vi "ziExample-Module-DAQ_triggerUtility.vi"() -> ()   [LabVIEW 2009]
doc: "Control a Zurich instrument device via the LabOne Labview API. \nRequirements: Zurich Instruments MFLI, HF2 or UHFLI \nThis example shows how to start a DAQ trigger module and retrieve the Data.\n\n© Zurich Instruments AG, www.zhinst.com"
uses:
  <instrlib>/Zurich Instruments LabOne/Public/Modules/ziTypeModEnum.ctl
  <instrlib>/Zurich Instruments LabOne/Public/Modules/ziModSetValueBinary.vi
  <instrlib>/Zurich Instruments LabOne/Public/Configure/ziSetValueDoubleArray.vi
  <instrlib>/Zurich Instruments LabOne/Public/Modules/ziModSetValueDouble.vi
  <instrlib>/Zurich Instruments LabOne/Public/Modules/ziModGetDoubleData.vi
  <instrlib>/Zurich Instruments LabOne/Public/Utility/ziTicksToS_vector.vi
  <instrlib>/Zurich Instruments LabOne/Public/Utility/ziTicksToS_single.vi
  <instrlib>/Zurich Instruments LabOne/Zurich Instruments LabOne.lvlib
panel:
  in  "beating":bool caption="Beating (needs MD/MF Option)"
  out "Slide":dbl(slide) scale=0.0..1.0
  in  "subscribe":string="demods/0/sample.R.avg"
  out "Grid DEMOD X":dbl[][](graph)
  out "Error Out":errorcluster
  in  "stop":bool
  in  "run":bool caption="Run"
  in  "TriggerModulSetup":T1={"holdoff/time"=0.2, "holdoff/count"=0.0, "delay"=-0.00125, "duration"=0.01, "pulse/min"=0.0, "pulse/max"=0.0, "type"=1, "edge"=1, "count"=5.0, "bits"=1.0, "bitmask"=1.0, "triggernode"="demods/0/sample.R", "bandwidth"=0.0, "hysteresis"=0.003, "level"=0.03, "grid/mode"=1.0, "grid/cols"=100, "grid/rows"=100, "grid/direction"=0.0, "grid/repetitions"=1.0} {"grid/direction" items=["Forward", "Reverse", "Bi-directional"]; "grid/mode" items=["OFF", "Nearest", "Linear"]; "level" format="%#_6p"; "hysteresis" format="%#_6p"; "bandwidth" format="%#_6p"; "edge" items=["positive"=1, "negative"=2, "both"=3]; "type" items=["edge"=1, "digital"=2, "pulse"=3, "tracking edge"=4, "HW Trigger"=6, "tracking pulse"=7]}
  out "Demod X":T2(graph)
  in  "Address":string="DEV"
  out "Selected Device":string
  # "ziExample-Module-DAQ_triggerUtility.vi\nRequirements: \n- HF2LI, UHFLI or MFLI \n- MD Option\nsee block diagram for VI description"
  # "Tested Instruments:\n- HF2LI\n- UHFLI\n- MFLI"
  # "Trigger Settings"
  # "edge/pulse/tracking edge/tracking pulse"
  # "only for tracking mode"
  # "digital"
  # "Horizontal"
  # "only for pulse/tracking pulse"
  # "only for pulse/tracking pulse"
  # "Grid Mode"
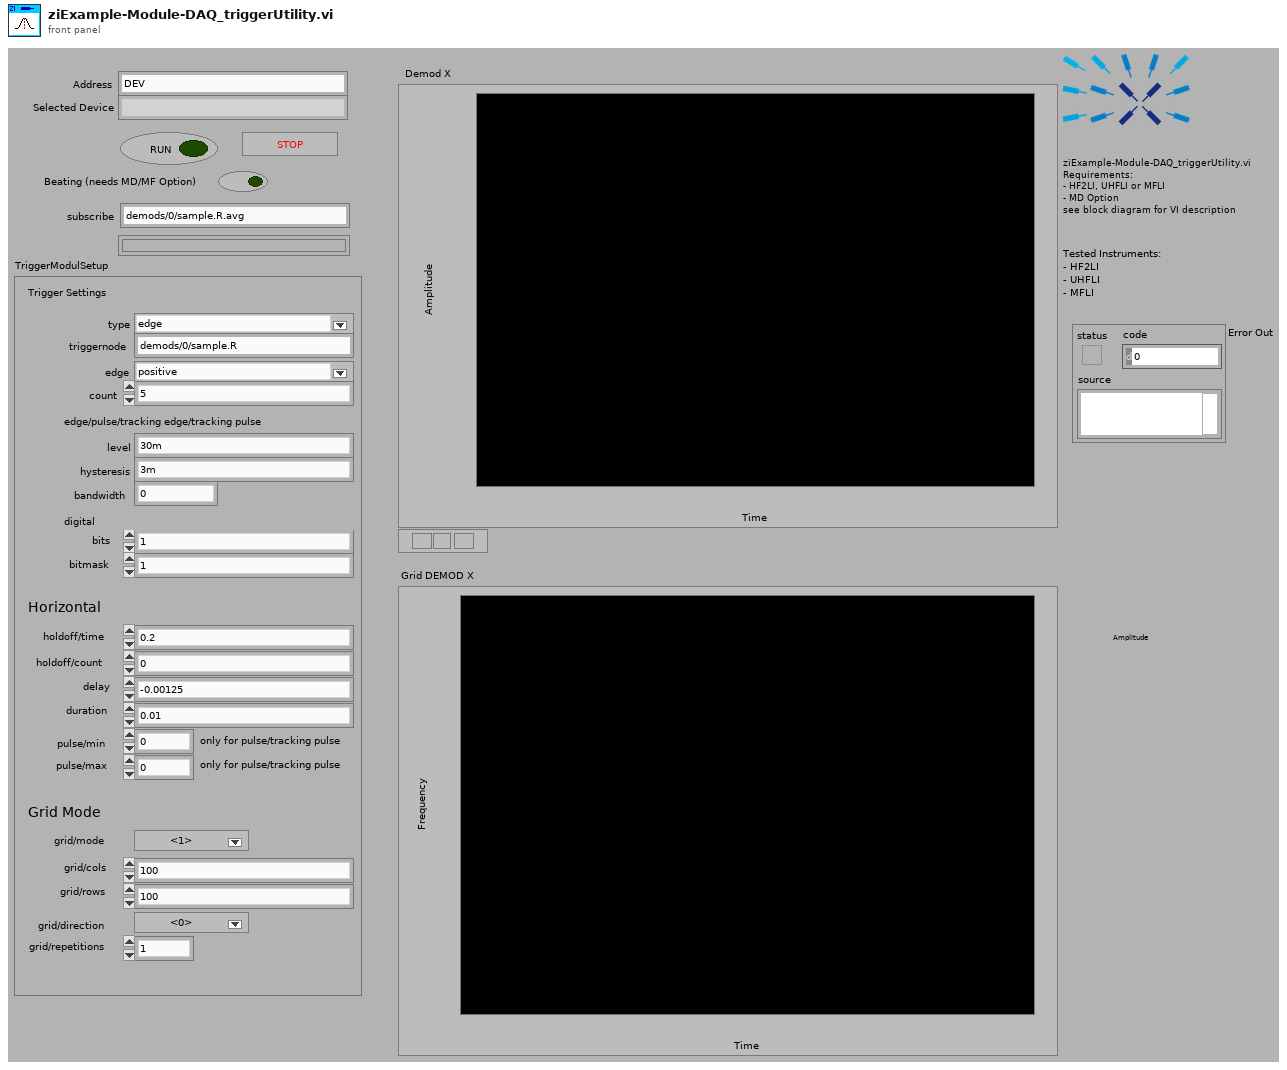
[diagram p1: front panel]
types:
  T1 = cluster{"holdoff/time":dbl, "holdoff/count":dbl, "delay":dbl, "duration":dbl, "pulse/min":dbl, "pulse/max":dbl, "type":u16, "edge":u16, "count":dbl, "bits":dbl, "bitmask":dbl, "triggernode":string, "bandwidth":dbl, "hysteresis":dbl, "level":dbl, "grid/mode":dbl, "grid/cols":u32, "grid/rows":u32, "grid/direction":dbl, "grid/repetitions":dbl}
  T2 = cluster{"Timestamp(s)":dbl[], "X (Vrms)":dbl[]}[]
  T3 = typedef "Zurich Instruments LabOne.lvlib/ziTypeModEnum.ctl" = u16
  T4 = typedef "Zurich Instruments LabOne.lvlib/ziTypeHandle.ctl" = cluster{"handleValid":bool, "Conn":u64, "Path Prefix":string, "Handle":u64, "Connected":bool, "Clockbase(s)":dbl}
  T5 = typedef "Zurich Instruments LabOne.lvlib/ziTypeModHandle.ctl" = cluster{"handleValid":bool, "Conn":u64, "ModHandle":u64, "moduleID":string, "Path Prefix":string}
  T6 = typedef "Zurich Instruments LabOne.lvlib/ziTypeModResults.ctl" = cluster{"PathArray":string[], "ValueType":T7, "NoOfResults":u64, "ziGenericHeader":T8[]}
  T7 = typedef "Zurich Instruments LabOne.lvlib/ziTypePollType.ctl" = enum16{"NONE", "DOUBLE_DATA", "INTEGER_DATA", "DEMOD_SAMPLE", "SCOPE_WAVE_HF2", "AUXIN_SAMPLE", "DIO_SAMPLE", "BYTE_ARRAY", "PWA_WAVE", "9", "10", "11", "12", "13", "14", "15", "TREE_CHANGE_DEPRI", "17", "ERROR", "19", "20", "21", "22", "23", "24", "25", "26", "27", "28", "29", "30", "31", "DOUBLE_DATA_TS", "INTEGER_DATA_TS", "34", "SCOPE_WAVE", "SCOPE_WAVE_EX", "37", "BYTE_ARRAY_TS", "39", "40", "41", "42", "43", "44", "45", "CNT_DATA", "47", "TREE_CHANGE", "49", "50", "51", "52", "53", "54", "55", "56", "57", "58", "59", "60", "61", "62", "63", "SWEEPER_DATA", "SPECTRUM_DATA", "ADVISOR_DATA", "VECTOR_DATA", "IMP_DATA"}
  T8 = typedef "Zurich Instruments LabOne.lvlib/ziTypeModGenericHeader.ctl" = cluster{"HeaderType":enum8{"HEADER_TYPE_NONE", "HEADER_TYPE_SWTRIGGER", "HEADER_TYPE_SWEEPER"}, "SampleFormat":u8, "SystemTime":timestamp, "CreatedTimeStamp":u64, "ChangedTimeStamp":u64, "Flags":u32, "ChunkSizeBytes":u64, "Name":string, "Status":u32, "GroupIndex":u32, "Color":u32, "ActiveRow":u32, "TriggerNumber":u64, "GridRows":u32, "GridCols":u32, "GridMode":u32, "GridOperation":u32, "GridDirection":u32, "GridRepetitions":u32, "GridColDelta":dbl, "GridColOffset":dbl, "GridRowDelta":dbl, "GridRowOffset":dbl, "Bandwidth":dbl, "Center":dbl, "Nenbw":dbl}
  T9 = typedef "Zurich Instruments LabOne.lvlib/ziTypeDoubleDataTSGrid.ctl" = cluster{"Timestamp (ticks)":u64[][], "Value":dbl[][]}
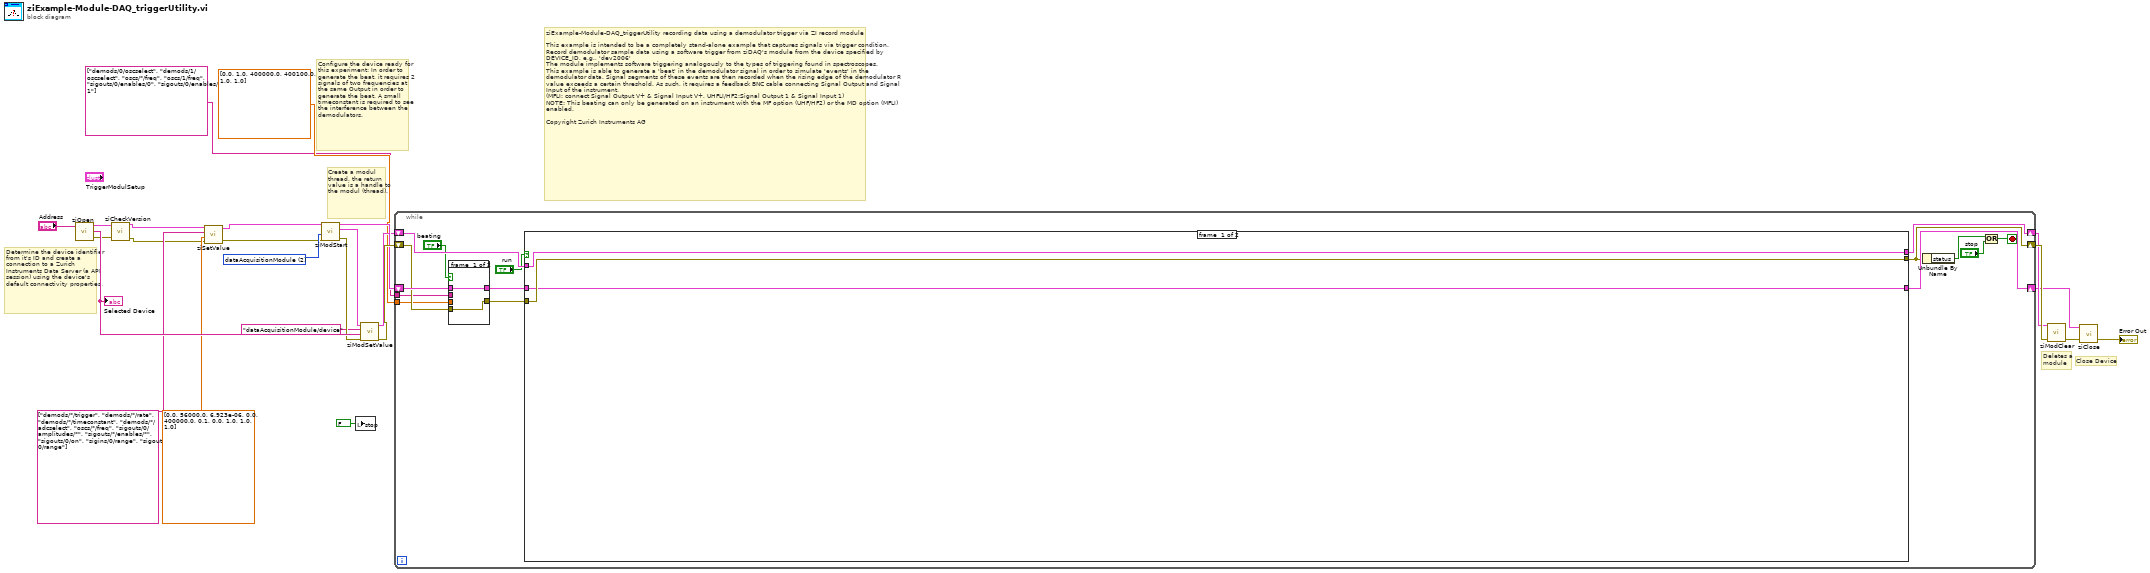
[diagram p0: block diagram]
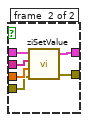
[diagram p2: hidden frame]
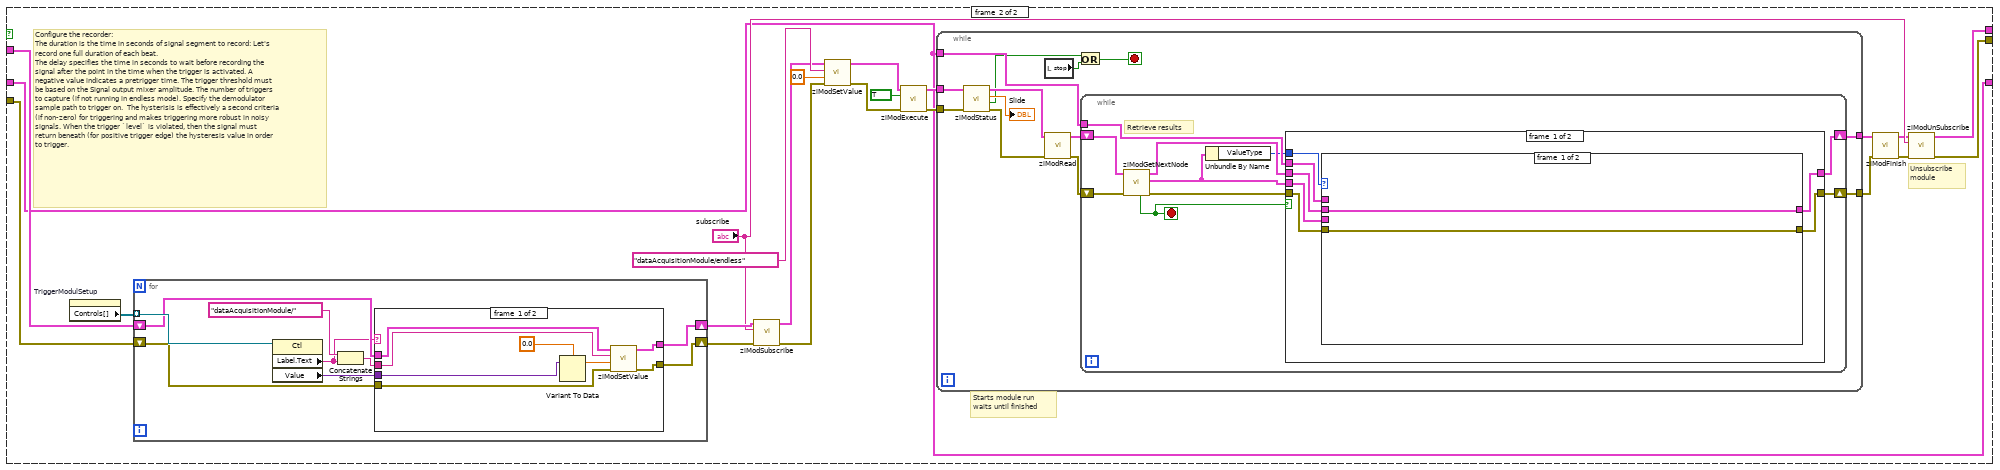
[diagram p3: hidden frame]
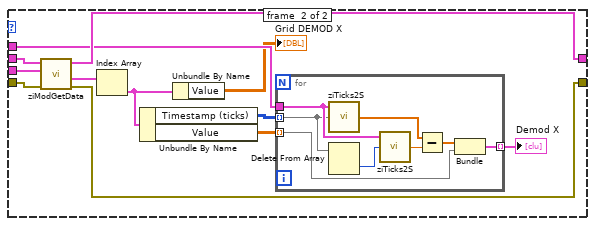
[diagram p4: hidden frame]
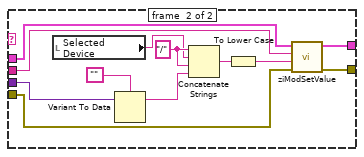
[diagram p6: hidden frame]
diagram:
  w5 = T3 2 items=["sweep", "scopeModule", "dataAcquisitionModule", "pidAdvisor", "awgModule", "impedanceModule", "multiDeviceSyncModule", "zoomFFT", "trigger", "deviceSettings", "record"] ("module Id")
  # "ziExample-Module-DAQ_triggerUtility recording data using a demodulator trigger via ZI record module\n\nThis example is intended to be a completely stand-alone example that captures signals via trigger condition. \nRecord demodulator sample data using a software trigger from ziDAQ's module from the device specified by DEVICE_ID, e.g., 'dev2006' \nThe module implements software triggering analogously to the types of triggering found in spectroscopes.\nThis example is able to generate a 'beat' in the demodulator signal in order to simulate 'events' in the demodulator data. Signal segments of these events are then recorded when the rising edge of the demodulator R value exceeds a certain threshold. As such, it requires a feedback BNC cable connecting Signal Output and Signal Input of the instrument. \n(MFLI: connect Signal Output V+ & Signal Input V+, UHFLI/HF2:Signal Output 1 & Signal Input 1)\nNOTE: This beating can only be generated on an instrument with the MF option (UHF/HF2) or the MD option (MFLI) enabled.\n\nCopyright Zurich Instruments AG"
  # "Configure the device ready for this experiment: In order to generate the beat, it requires 2 signals of two frequencies at the same Output in order to generate the beat. A small timeconstant is required to see the interference between the demodulators."
  # "Deletes a\nmodule"
  # "Create a modul thread, the return value is a handle to the modul (thread)."
  # "Close Device"
  # "Determine the device identifier from it's ID and create a connection to a Zurich Instruments Data Server (a API session) using the device's default connectivity properties."
  n1 = call <instrlib>:"ziOpen.vi"("Address"="Address") -> ("Error Out"=w8:errorcluster, "Selected Device"=w24:string, "HandleOut"=w9:T4)  [unwired: 1 in, 2 out]
  "Selected Device" <- w24
  n2 = call <instrlib>:"ziCheckVersion.vi"("Handle In"=w9, "Error In"=w8) -> ("Handle Out"=w7:T4, "Error Out"=w6:errorcluster)  [unwired: 11 in, 1 out]
  n3 = call-poly <instrlib>:"ziSetValue.vi"("Error In"=w6, "Values"=dbl[] [0.0, 56000.0, 6.923e-06, 0.0, 400000.0, 0.1, 0.0, 1.0, 1.0, 1.0], "Paths"=string[] ["demods/*/trigger", "demods/*/rate", "demods/*/timeconstant", "demods/*/adcselect", "oscs/*/freq", "sigouts/0/amplitudes/*", "sigouts/*/enables/*", "sigouts/0/on", "sigins/0/range", "sigouts/0/range"], "Handle In"=w7) -> ("Error Out"=w4:errorcluster, "Handle Out"=w3:T4)  [unwired: 1 in]
  n4 = call <instrlib>:"ziModStart.vi"("Error In"=w4, "module Id"=w5, "Handle In"=w3) -> ("Error Out"=w22:errorcluster, "ModHandle Out"=w23:T5, "Handle Out"=w18:T4)  [unwired: 6 in]
  n5 = local write "stop"(FALSE ("stop")) -> ()
  n6 = call-poly <instrlib>:"ziModSetValue.vi"("Error In"=w22, "Data"=w24, "Path"="dataAcquisitionModule/device", "ModHandle In"=w23) -> ("Error Out"=w19:errorcluster, "ModHandle Out"=w14:T5)  [unwired: 6 in]
  n7 = while {
    shift-right: [w38] -> w16
    shift-left: w14 -> [w40]
    shift-right: [w33] -> w17
    shift-left: w19 -> [w30]
    shift-right: [w37] -> w10
    shift-left: w18 -> [w31]
    tunnel: dbl[] [0.0, 1.0, 400000.0, 400100.0, 1.0, 1.0] -> [w28]
    tunnel: string[] ["demods/0/oscselect", "demods/1/oscselect", "oscs/*/freq", "oscs/1/freq", "sigouts/0/enables/0", "sigouts/0/enables/1"] -> [w27]
    stop <- w34 stop-if-true
    n8 = case shown="False" "beating" {
      tunnel: [w42 w48] -> w32
      tunnel: [w41 w47] -> w29
      tunnel: w27 -> [_ w46]
      tunnel: w28 -> [_ w45]
      tunnel: w31 -> [w42 w44]
      tunnel: w30 -> [w41 w43]
      frame #0 {
      }
      frame #1 {
        n9 = call-poly <instrlib>:"ziSetValue.vi"("Error In"=w43, "Values"=w45, "Paths"=w46, "Handle In"=w44) -> ("Error Out"=w47:errorcluster, "Handle Out"=w48:T4)  [unwired: 1 in]
      }
    }
    n10 = case shown="True" "run" {
      tunnel: [w50 w64] -> w38
      tunnel: [w51 w54] -> w33
      tunnel: w32 -> [w49 w55]
      tunnel: w40 -> [w50 w68]
      tunnel: w29 -> [w51 w67]
      tunnel: [w49 w55] -> w37
      frame #0 {
      }
      frame #1 {
        # "Unsubscribe\nmodule"
        # "Starts module run\nwaits until finished"
        # "Configure the recorder:\nThe duration is the time in seconds of signal segment to record: Let's record one full duration of each beat.\nThe delay specifies the time in seconds to wait before recording the signal after the point in the time when the trigger is activated. A negative value indicates a pretrigger time. The trigger threshold must be based on the Signal output mixer amplitude. The number of triggers to capture (if not running in endless mode). Specify the demodulator sample path to trigger on.  The hysterisis is effectively a second criteria (if non-zero) for triggering and makes triggering more robust in noisy signals. When the trigger `level` is violated, then the signal must return beneath (for positive trigger edge) the hysteresis value in order to trigger."
        n11 = property on="TriggerModulSetup" class="Clust (strict)"() -> ("Controls[]"=w71:refnum<vi>[])  [unwired: 2 in, 2 out]
        n12 = for {
          tunnel: w71 -> [w136] mode=indexing
          shift-right: [w133] -> w69
          shift-left: w67 -> [w131]
          shift-right: [w134] -> w70
          shift-left: w68 -> [w132]
          n13 = property class="Ctl"(reference=w136) -> ("Label.Text"=w129:string, "Value"=w128:variant)  [unwired: 1 in, 2 out]
          n14 = Concatenate Strings("dataAcquisitionModule/" ("string"), w129) -> (w130:string)
          n15 = case shown="\"triggernode\"" w129 {
            tunnel: w130 -> [w137 w150]
            tunnel: w128 -> [w144 w155]
            tunnel: [w141 w154] -> w134
            tunnel: [w140 w153] -> w133
            tunnel: w132 -> [w142 w152]
            tunnel: w131 -> [w139 w151]
            frame #0 {
              n16 = Variant To Data(Variant=w144, type=0.0) -> (data=w138:dbl)  [unwired: 1 in, 1 out]
              n17 = call-poly <instrlib>:"ziModSetValue.vi"("Error In"=w139, "Value"=w138, "Path"=w137, "ModHandle In"=w142) -> ("Error Out"=w140:errorcluster, "ModHandle Out"=w141:T5)  [unwired: 6 in]
            }
            frame #1 {
              w149 = "/"
              n18 = local read "Selected Device"() -> (w148:string)
              n19 = Variant To Data(Variant=w155, type="") -> (data=w147:string)  [unwired: 1 in, 1 out]
              n20 = Concatenate Strings(w149, w148, w149, w147) -> (w146:string)
              n21 = To Lower Case(string=w146) -> (all lower case string=w145:string)
              n22 = call-poly <instrlib>:"ziModSetValue.vi"("Error In"=w151, "Data"=w145, "Path"=w150, "ModHandle In"=w152) -> ("Error Out"=w153:errorcluster, "ModHandle Out"=w154:T5)  [unwired: 6 in]
            }
          }
        }
        n23 = call <instrlib>:"ziModSubscribe.vi"("Error In"=w69, "Path"="subscribe", "ModHandle In"=w70) -> ("Error Out"=w53:errorcluster, "ModHandle Out"=w52:T5)  [unwired: 6 in]
        n24 = call-poly <instrlib>:"ziModSetValue.vi"("Error In"=w53, "Value"=0.0, "Path"="dataAcquisitionModule/endless", "ModHandle In"=w52) -> ("Error Out"=w65:errorcluster, "ModHandle Out"=w66:T5)  [unwired: 6 in]
        n25 = call <instrlib>:"ziModExecute.vi"("Error In"=w65, "Modal (F)"=TRUE, "ziModHandle In"=w66) -> ("Error Out"=w60:errorcluster, "ziModHandle Out"=w61:T5)  [unwired: 5 in, 1 out]
        n26 = while {
          tunnel: w55 -> [w86]
          tunnel: w61 -> [w81]
          tunnel: w60 -> [w80]
          tunnel: [w79] -> w58
          tunnel: [w78] -> w57
          stop <- w74 stop-if-true
          n27 = call <instrlib>:"ziModStatus.vi"("Error In"=w80, "ModHandle IN"=w81) -> ("Error Out"=w82:errorcluster, "Finished?"=w75:bool, "Progress (unity)"=→"Slide":dbl, "ModHandle Out"=w83:T5)  [unwired: 5 in]
          n28 = local read "stop"() -> (w76:bool)
          n29 = call <instrlib>:"ziModRead.vi"("error in"=w82, "ziModHandle In"=w83) -> ("error out"=w85:errorcluster, "ziModHandle Out"=w84:T5)  [unwired: 8 in]
          n30 = Or(x=w75, y=w76) -> (x .or. y?=w74:bool)
          n31 = while {
            shift-right: [w91] -> w78
            shift-left: w84 -> [w95]
            shift-right: [w92] -> w79
            shift-left: w85 -> [w96]
            tunnel: w86 -> [w90]
            stop <- w89 stop-if-true
            # "Retrieve results"
            n32 = call <instrlib>:"ziModGetNextNode.vi"("Error In"=w96, "ModHandle In"=w95) -> ("Error Out"=w93:errorcluster, "ModResults"=w87:T6, "ModHandle Out"=w94:T5, "NoData"=w89:bool)  [unwired: 6 in]
            n33 = Unbundle By Name(w87) -> ("ValueType"=w88:T7)
            n34 = case shown="False" w89 {
              tunnel: w87 -> [w103 _]
              tunnel: w94 -> [w102 w127]
              tunnel: w93 -> [w101 w126]
              tunnel: [w100 w126] -> w92
              tunnel: [w99 w127] -> w91
              tunnel: w88 -> [w98 _]
              tunnel: w90 -> [w97 _]
              frame #0 {
                n35 = case shown="\"DOUBLE_DATA_TS\"" w98 {
                  tunnel: w102 -> [w105 w110]
                  tunnel: w103 -> [_ w109]
                  tunnel: w101 -> [w104 w114]
                  tunnel: [w104 w115] -> w100
                  tunnel: [w105 w117] -> w99
                  tunnel: w97 -> [_ w116]
                  frame #0 {
                  }
                  frame #1 {
                    n36 = call-poly <instrlib>:"ziModGetData.vi"("Error In"=w114, "ModResults"=w109, "ModHandle In"=w110) -> ("Error Out"=w115:errorcluster, "DoubleSampleGrid"=w113:T9[], "ModHandle Out"=w117:T5)  [unwired: 4 in, 2 out]
                    n37 = Index Array(array=w113) -> (element=w108:T9)  [unwired: 1 in]
                    n38 = Unbundle By Name(w108) -> ("Timestamp (ticks)"=w107:u64[][], "Value"=w106:dbl[][])
                    n39 = Unbundle By Name(w108) -> ("Value"=→"Grid DEMOD X":dbl[][])
                    n40 = for {
                      tunnel: [w125] -> w111 mode=indexing
                      tunnel: w116 -> [w124]
                      tunnel: w107 -> [w119] mode=indexing
                      tunnel: w106 -> [w120] mode=indexing
                      n41 = call-poly <instrlib>:"ziTicks2S.vi"("Timestamp (ticks)"=w119, "Handle In"=w124) -> ("Timestamp(s)"=w122:dbl[])  [unwired: 1 in, 2 out]
                      n42 = Delete From Array(array=w119) -> (deleted portion=w118:u64)  [unwired: 2 in, 1 out]
                      n43 = call-poly <instrlib>:"ziTicks2S.vi"("Timestamp(ticks)"=w118, "Handle In"=w124) -> ("Timestamp(s)"=w123:dbl)  [unwired: 1 in, 2 out]
                      n44 = Subtract(x=w122, y=w123) -> (x-y=w121:dbl[])
                      n45 = Bundle(w121, "Value"=w120) -> (w125:cluster{dbl[], "Value":dbl[]})  [unwired: 1 in]
                    }
                    "Demod X" <- w111
                  }
                }
              }
              frame #1 {
              }
            }
          }
        }
        n46 = call <instrlib>:"ziModFinish.vi"("Error In"=w58, "ziModHandle In"=w57) -> ("Error Out"=w59:errorcluster, "ziModHandle Out"=w56:T5)  [unwired: 7 in]
        n47 = call <instrlib>:"ziModUnSubscribe.vi"("Error In"=w59, "Path (\"/\")"="subscribe", "ModHandle In"=w56) -> ("Error Out"=w54:errorcluster, "ModHandle Out"=w64:T5)  [unwired: 7 in]
      }
    }
    n48 = Unbundle By Name(w33) -> ("status"=w36:bool)
    n49 = Or(x=w36, y="stop") -> (x .or. y?=w34:bool)
  }
  n50 = call <instrlib>:"ziModClear.vi"("Error In"=w17, "ziModHandle In"=w16) -> ("Error Out"=w25:errorcluster)  [unwired: 7 in, 1 out]
  n51 = call <instrlib>:"ziClose.vi"("Error In"=w25, "Handle In"=w10) -> ("Error Out"=→"Error Out":errorcluster)  [unwired: 2 in, 1 out]
